vi "FTDI_DX22_clear_sys_flags.vi"(8 "error in (no error)":errorcluster, 11 "Handle":u64) -> (0 "error out":errorcluster, 3 "Handle out":u64)   [LabVIEW 2019]
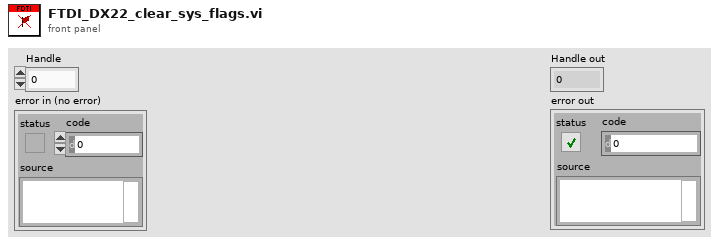
[diagram p1: front panel]
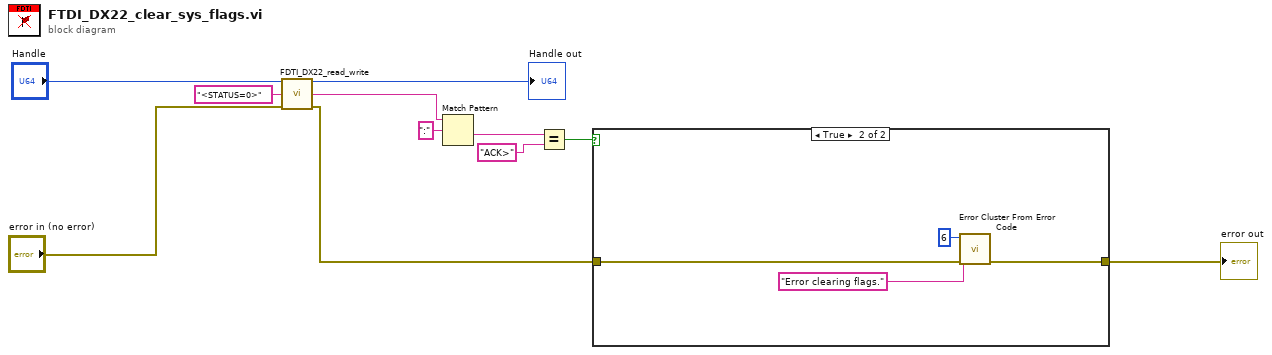
[diagram p0: block diagram]
diagram:
  n1 = call "FDTI_DX22_read_write.vi"("Handle"="Handle", "Write string"="<STATUS=0>", "error in (no error)"="error in (no error)") -> ("Handle out"=→"Handle out":u64, "Read Data"=w7:string, "error out"=w2:errorcluster)  [unwired: 10 in]
  n2 = Match Pattern(string=w7, regular expression=":") -> (after substring=w5:string)  [unwired: 1 in, 3 out]
  n3 = Equal?(x=w5, y="ACK>") -> (x = y?=w3:bool)
  n4 = case shown="True" w3 {
    tunnel: w2 -> [w12 w14]
    tunnel: [w12 w13] -> w1
    frame False {
    }
    frame True {
      n5 = call <vilib>:"Error Cluster From Error Code.vi"("error in (no error)"=w14, "error message (\"\")"="Error clearing flags." ("error message (\"\")"), "error code (0)"=6) -> ("error out"=w13:errorcluster)  [unwired: 6 in]
    }
  }
  "error out" <- w1
